vi "SubMotores.vi"() -> ()   [LabVIEW 2012]
doc: "An example using two servos with the LabVIEW Interface for Arduino."
uses:
  <vilib>/LabVIEW Interface for Arduino/LabVIEW Interface for Arduino.lvlib
panel:
  in  "Stop":bool
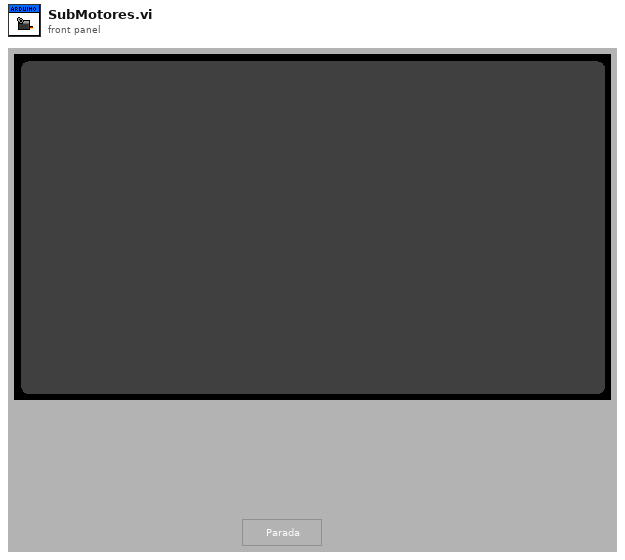
[diagram p1: front panel]
types:
  T1 = typedef "LabVIEW Interface for Arduino.lvlib/Arduino Resource.ctl" = cluster{"VISA resource":refnum<visa-resource-name>, "Board Type":T2, "Connection Type":enum8{"USB / Serial"}, "Bytes Per Packet (15)":u8}
  T2 = typedef "LabVIEW Interface for Arduino.lvlib/Board Type.ctl" = enum16{"Uno", "Dimuelanove w/Atmega 328", "Mega 2560"}
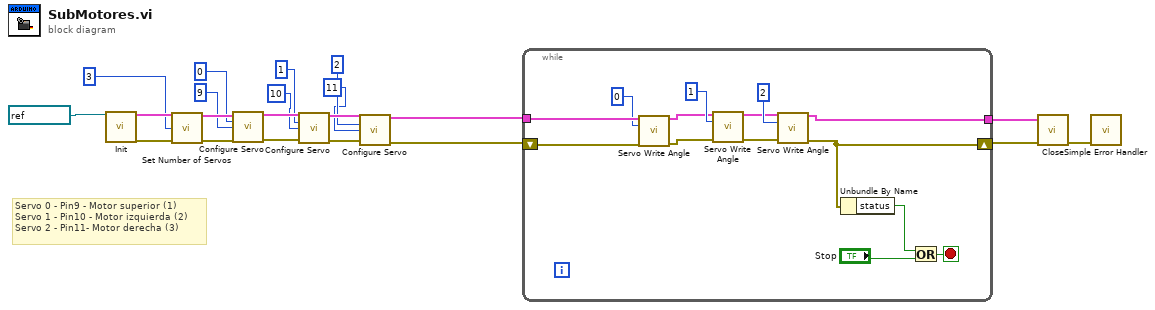
[diagram p0: block diagram]
diagram:
  # "Servo 0 - Pin9 - Motor superior (1)\nServo 1 - Pin10 - Motor izquierda (2)\nServo 2 - Pin11- Motor derecha (3)"
  n1 = call <vilib>:"Init.vi"("VISA resource"=refnum<visa-resource-name> "COM4") -> ("Arduino Resource"=w12:T1, "error out"=w21:errorcluster)  [unwired: 17 in]
  n2 = call <vilib>:"Set Number of Servos.vi"("Arduino Resource"=w12, "Number Of Servos (1)"=u8 3 ("Servo Number"), "error in"=w21) -> ("Arduino Resource"=w20:T1, "error out"=w19:errorcluster)  [unwired: 11 in]
  n3 = call <vilib>:"Configure Servo.vi"("Arduino Resource"=w20, "Servo Number (0)"=u8 0 ("Servo Number"), "DIO Pin (2)"=u8 9 ("Servo Number"), "error in"=w19) -> ("Arduino Resource"=w7:T1, "error out"=w10:errorcluster)  [unwired: 10 in]
  n4 = call <vilib>:"Configure Servo.vi"("Arduino Resource"=w7, "Servo Number (0)"=u8 1 ("Servo Number"), "DIO Pin (2)"=u8 10 ("Servo Number"), "error in"=w10) -> ("Arduino Resource"=w6:T1, "error out"=w9:errorcluster)  [unwired: 10 in]
  n5 = call <vilib>:"Configure Servo.vi"("Arduino Resource"=w6, "Servo Number (0)"=u8 2 ("Servo Number"), "DIO Pin (2)"=u8 11 ("Servo Number"), "error in"=w9) -> ("Arduino Resource"=w5:T1, "error out"=w8:errorcluster)  [unwired: 10 in]
  n6 = while {
    tunnel: w5 -> [w35]
    tunnel: [w25] -> w15
    shift-right: [w22] -> w16
    shift-left: w8 -> [w34]
    stop <- w33 stop-if-true
    n7 = call <vilib>:"Servo Write Angle.vi"("Arduino Resource"=w35, "Servo Number"=u8 0, "error in"=w34) -> ("Arduino Resource"=w27:T1, "error out"=w24:errorcluster)  [unwired: 11 in]
    n8 = call <vilib>:"Servo Write Angle.vi"("Arduino Resource"=w27, "Servo Number"=u8 1, "error in"=w24) -> ("Arduino Resource"=w26:T1, "error out"=w23:errorcluster)  [unwired: 11 in]
    n9 = call <vilib>:"Servo Write Angle.vi"("Arduino Resource"=w26, "Servo Number"=u8 2, "error in"=w23) -> ("Arduino Resource"=w25:T1, "error out"=w22:errorcluster)  [unwired: 11 in]
    n10 = Unbundle By Name(w22) -> ("status"=w32:bool)
    n11 = Or(x=w32, y="Stop") -> (x .or. y?=w33:bool)
  }
  n12 = call <vilib>:"Close.vi"("Arduino Resource"=w15, "error in"=w16) -> ("error out"=w13:errorcluster)  [unwired: 13 in]
  n13 = call <vilib>:"Simple Error Handler.vi"("error in (no error)"=w13) -> ()  [unwired: 4 in, 5 out]
